vi "BdcstTrigger.vi"(8 "error in (no error)":errorcluster, 9 "Trigger":T1={"Coupling"=enum."AC", "Holdoff"=0.0, "Level"=0.0, "Slope"=enum."Positive", "Source"="", "Type"=enum."Edge"}, 10 "ModuleID":i32) -> (0 "error out":errorcluster)   [LabVIEW 2018, in "ScopePlugins.lvlib"]
uses:
  ScopePlugins.lvlib
  TypeDefs/Trigger.ctl
  ScopeShared/clEventType.ctl
  ScopeShared/ScopeShared.lvlib
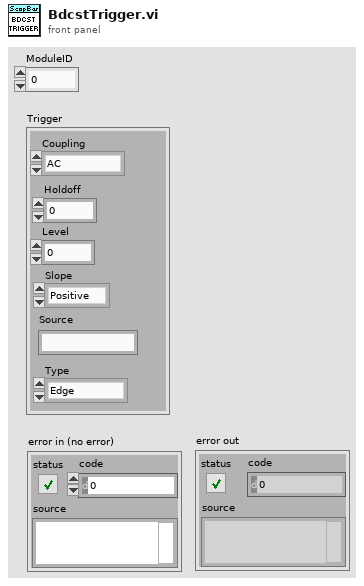
[diagram p1: front panel]
types:
  T1 = typedef "ScopePlugins.lvlib/Trigger.ctl" = cluster{"Coupling":enum16{"AC", "DC", "LF Reject", "HF Reject", "Noise Reject"}, "Holdoff":dbl, "Level":dbl, "Slope":enum16{"Negative", "Positive"}, "Source":string, "Type":enum16{"Edge", "Width", "Runt", "Glitch", "TV", "Immediate", "AC Line"}}
  T2 = typedef "ScopeShared.lvlib/clEventType.ctl" = cluster{"ModuleID":i32, "Data":variant}
  T3 = typedef "ScopeShared.lvlib/clBroadcastEvents.ctl" = cluster{"DidInit":refnum<user-event>, "StatusUpdate":refnum<user-event>, "ErrorReport":refnum<user-event>, "DidStop":refnum<user-event>, "PathToINI":refnum<user-event>, "Handle":refnum<user-event>, "Model":refnum<user-event>, "Channels":refnum<user-event>, "Acquisition":refnum<user-event>, "Trigger":refnum<user-event>, "ExtAcquisition":refnum<user-event>, "Waveform":refnum<user-event>}
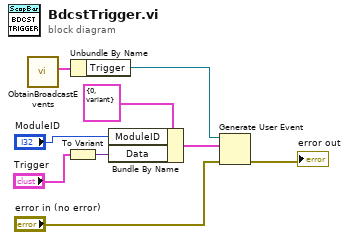
[diagram p0: block diagram]
diagram:
  n1 = call "ObtainBroadcastEvents.vi"() -> ("clBroadcastEvents"=w9:T3)  [unwired: 10 in, 1 out]
  n2 = To Variant(anything="Trigger") -> (Variant=w5:variant)
  n3 = Unbundle By Name(w9) -> ("Trigger"=w8:refnum<user-event>)
  n4 = Bundle By Name(cluster=T2 {"ModuleID"=0, "Data"=variant} ("clEventType"), "ModuleID"="ModuleID", "Data"=w5) -> (w2:T2)
  n5 = Generate User Event(user event=w8, event data cluster=w2, error in="error in (no error)") -> (error out=→"error out":errorcluster)  [unwired: 1 in, 1 out]
